vi "NewPort_PM_cmd-query_NAME(SubVI).vi"(0 "Dual: CH_1 \nLambda (nm)":i32, 1 "Pick Single CH \nCH1(F)\nCH2(T)":bool, 2 "Set Lambda\nSingle CH(F)\nDual CHs(T)":bool, 3 "Read Power\nSingle CH(F)\nDual CHs(T)":bool, 5 "Dual: CH_2\nLambda (nm)":i32, 9 "Single: CH\nLambda (nm)":i32, 11 "error in (no error)":errorcluster) -> (4 "Set Lambda (nm)":string, 8 "Read Power (W)":string, 15 "error out":errorcluster)   [LabVIEW 2017]
panel:
  out "Set Lambda_Single CH":string
  out "Set Lambda_Dual CH":string
  out "Read Power (W)_Single CH":string
  out "Read Power (W)_Dual CH":string
  # "Inputs"
  # "Outputs"
  # "Syntax Check"
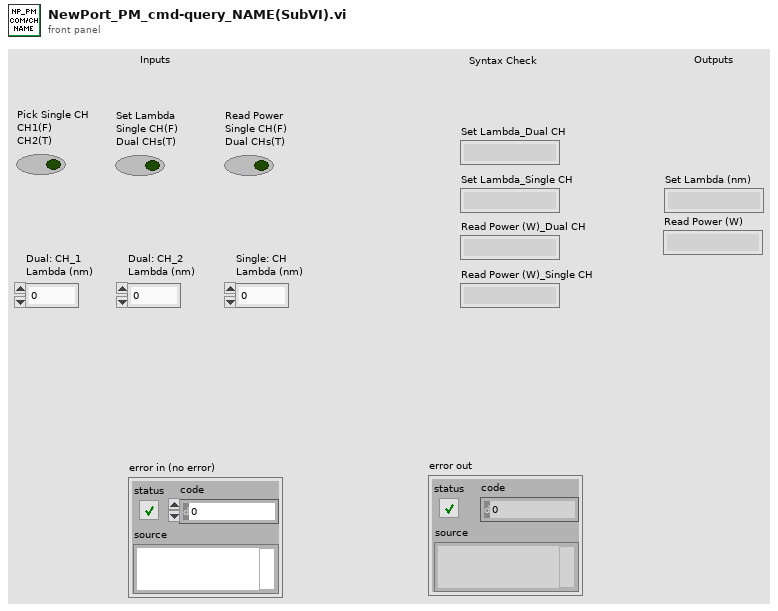
[diagram p1: front panel]
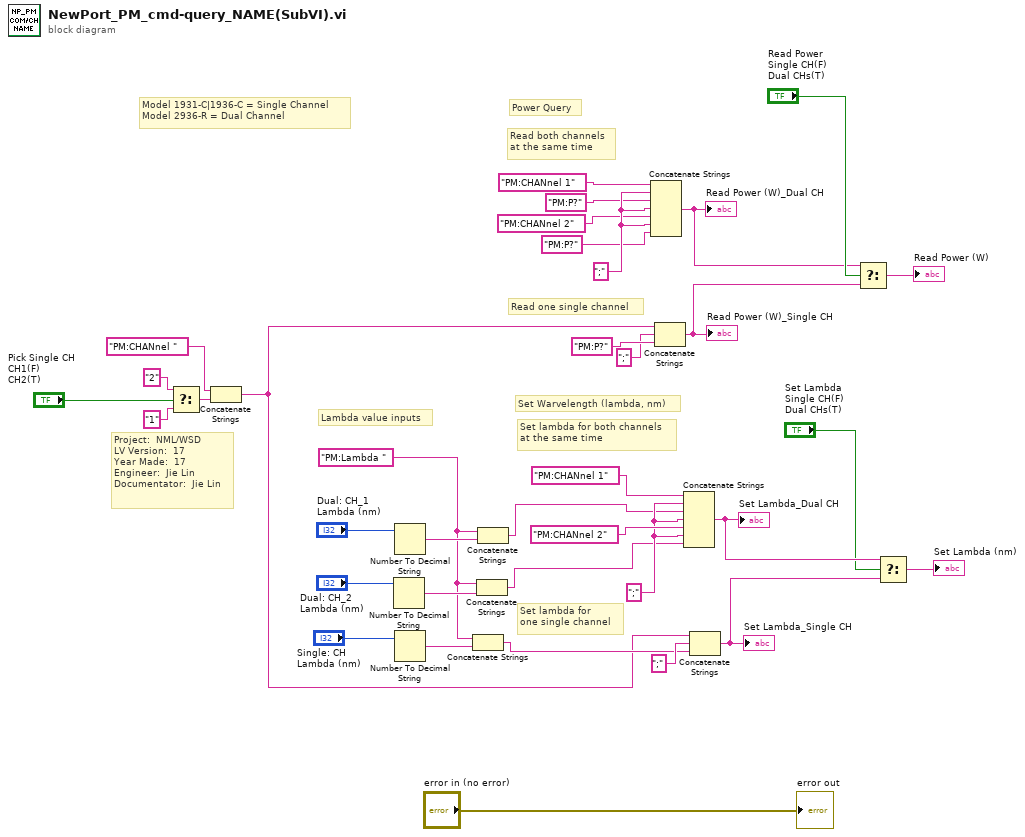
[diagram p0: block diagram]
diagram:
  w24 = ";" ("cmd")
  w25 = ";" ("cmd")
  w29 = "PM:Lambda " ("cmd")
  # "Project:  NML/WSD \nLV Version:  17\nYear Made:  17\nEngineer:  Jie Lin\nDocumentator:  Jie Lin"
  # "Model 1931-C|1936-C = Single Channel\nModel 2936-R = Dual Channel"
  # "Lambda value inputs"
  # "Set lambda for\none single channel"
  # "Set lambda for both channels\nat the same time"
  # "Read one single channel"
  # "Read both channels\nat the same time"
  # "Set Warvelength (lambda, nm)"
  # "Power Query"
  n1 = Select(t="2" ("cmd"), s="Pick Single CH \nCH1(F)\nCH2(T)", f="1" ("cmd")) -> (s? t:f=w13:string)
  n2 = Concatenate Strings("PM:CHANnel " ("cmd"), w13) -> (w5:string)
  n3 = Number To Decimal String(number="Dual: CH_2\nLambda (nm)") -> (decimal integer string=w30:string)  [unwired: 1 in]
  n4 = Number To Decimal String(number="Dual: CH_1 \nLambda (nm)") -> (decimal integer string=w31:string)  [unwired: 1 in]
  n5 = Number To Decimal String(number="Single: CH\nLambda (nm)") -> (decimal integer string=w28:string)  [unwired: 1 in]
  n6 = Concatenate Strings(w29, w28) -> (w18:string)
  n7 = Concatenate Strings(w29, w30) -> (w16:string)
  n8 = Concatenate Strings(w29, w31) -> (w17:string)
  n9 = Concatenate Strings("PM:CHANnel 1" ("cmd"), w24, "PM:P?" ("cmd"), w24, "PM:CHANnel 2" ("cmd"), w24, "PM:P?" ("cmd")) -> (w2:string)
  "Read Power (W)_Dual CH" <- w2
  n10 = Concatenate Strings(w5, ";" ("cmd"), "PM:P?" ("cmd")) -> (w1:string)
  "Read Power (W)_Single CH" <- w1
  n11 = Concatenate Strings("PM:CHANnel 1" ("cmd"), w25, w17, w25, "PM:CHANnel 2" ("cmd"), w25, w16) -> (w9:string)
  "Set Lambda_Dual CH" <- w9
  n12 = Concatenate Strings(w5, ";" ("cmd"), w18) -> (w8:string)
  "Set Lambda_Single CH" <- w8
  n13 = Select(t=w2, s="Read Power\nSingle CH(F)\nDual CHs(T)", f=w1) -> (s? t:f=→"Read Power (W)":string)
  n14 = Select(t=w9, s="Set Lambda\nSingle CH(F)\nDual CHs(T)", f=w8) -> (s? t:f=→"Set Lambda (nm)":string)
  "error out" <- "error in (no error)"
